vi "gyro_hand_and_boat_sync_test.vi"() -> ()   [LabVIEW 2017]
panel:
  out "kéz acc SNR":dbl
  out "hajó acc SNR":dbl
  out "hajó gyro SNR":dbl
  out "kéz gyro SNR":dbl
  out "hajó gyro Csapásszám [stroke/min]":dbl
  out "kéz gyro Csapásszám [stroke/min]":dbl
  out "kéz acc Csapásszám [stroke/min]":dbl
  out "hajó acc Csapásszám [stroke/min]":dbl
  in  "file path2 (use dialog)":path
  in  "file path1 (use dialog)":path
  out "Angular Velocity Graph":waveform(dbl)[](graph)
  out "Acceleration Graph":waveform(dbl)[](graph)
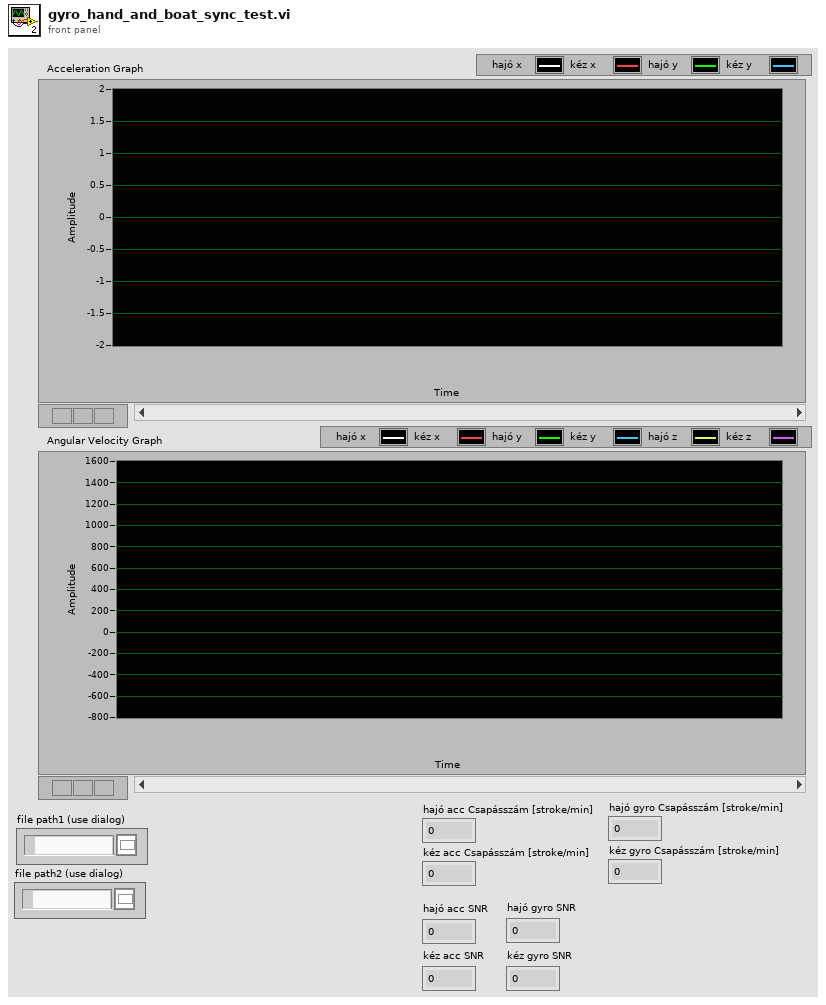
[diagram p1: front panel]
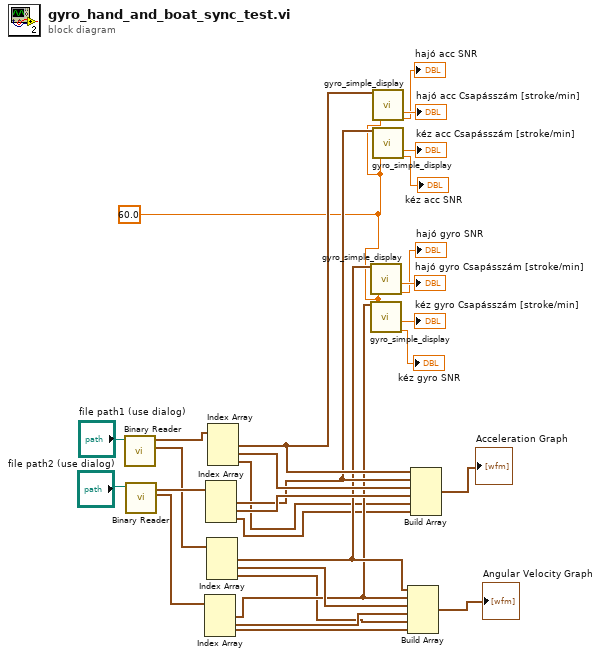
[diagram p0: block diagram]
diagram:
  w5 = 60.0 ("end")
  n1 = call "Binary Reader.vi"("file path (use dialog)"="file path1 (use dialog)") -> ("Angular Velocity"=w15:waveform(dbl)[], "Acceleration"=w26:waveform(dbl)[])  [unwired: 8 in, 1 out]
  n2 = call "Binary Reader.vi"("file path (use dialog)"="file path2 (use dialog)") -> ("Angular Velocity"=w14:waveform(dbl)[], "Acceleration"=w25:waveform(dbl)[])  [unwired: 8 in, 1 out]
  n3 = Index Array(array=w14) -> (element #1=w16:waveform(dbl), element #2=w23:waveform(dbl), element #3=w1:waveform(dbl))  [unwired: 3 in]
  n4 = Index Array(array=w25) -> (element #1=w18:waveform(dbl), element #2=w20:waveform(dbl), element #3=w3:waveform(dbl))  [unwired: 3 in]
  n5 = Index Array(array=w15) -> (element #1=w17:waveform(dbl), element #2=w24:waveform(dbl), element #3=w2:waveform(dbl))  [unwired: 3 in]
  n6 = Index Array(array=w26) -> (element #1=w19:waveform(dbl), element #2=w21:waveform(dbl), element #3=w4:waveform(dbl))  [unwired: 3 in]
  n7 = call "gyro_simple_display.vi"("waveform"=w17, "end"=w5) -> ("Csapásszám [stroke/min]"=→"hajó gyro Csapásszám [stroke/min]":dbl, "SNR"=→"hajó gyro SNR":dbl)  [unwired: 12 in, 4 out]
  n8 = call "gyro_simple_display.vi"("waveform"=w16, "end"=w5) -> ("Csapásszám [stroke/min]"=→"kéz gyro Csapásszám [stroke/min]":dbl, "SNR"=→"kéz gyro SNR":dbl)  [unwired: 12 in, 4 out]
  n9 = call "gyro_simple_display.vi"("waveform"=w19, "end"=w5) -> ("Csapásszám [stroke/min]"=→"hajó acc Csapásszám [stroke/min]":dbl, "SNR"=→"hajó acc SNR":dbl)  [unwired: 12 in, 4 out]
  n10 = call "gyro_simple_display.vi"("waveform"=w18, "end"=w5) -> ("Csapásszám [stroke/min]"=→"kéz acc Csapásszám [stroke/min]":dbl, "SNR"=→"kéz acc SNR":dbl)  [unwired: 12 in, 4 out]
  n11 = Build Array(w17, w16, w24, w23, w2, w1) -> (→"Angular Velocity Graph":waveform(dbl)[])
  n12 = Build Array(w19, w18, w21, w20, w4, w3) -> (→"Acceleration Graph":waveform(dbl)[])
